vi "sCOMS Trigger.vi"(11 "In":waveform(dbl)) -> (3 "Out":waveform(dbl))   [LabVIEW 2018]
uses:
  <vilib>/measure/NI_MABase.lvlib
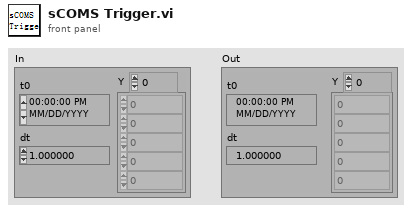
[diagram p1: front panel]
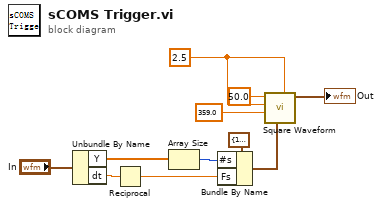
[diagram p0: block diagram]
diagram:
  w1 = 2.5 ("offset")
  n1 = Unbundle By Name("In") -> ("Y"=w4:dbl[], "dt"=w8:dbl)
  n2 = Reciprocal(x=w8) -> (1/x=w9:dbl)
  n3 = Array Size(array=w4) -> (size(s)=w7:i32)
  n4 = Bundle By Name(cluster=cluster{"Fs":dbl, "#s":dbl} {"Fs"=1000.0, "#s"=1000.0} ("sampling info"), "#s"=w7, "Fs"=w9) -> (w6:cluster{"Fs":dbl, "#s":dbl})
  n5 = call <vilib>:"Square Waveform.vi"("offset"=w1, "sampling info"=w6, "phase"=359.0, "amplitude"=w1, "frequency"=50.0) -> ("signal out"=→"Out":waveform(dbl))  [unwired: 5 in, 1 out]
